vi "ard write read.vi"(8 "error in (no error)":errorcluster, 11 "VISA Refnum in":refnum<visa-resource-name>) -> (0 "error out":errorcluster, 2 "Numeric":dbl, 3 "VISA Refnum out":refnum<visa-resource-name>)   [LabVIEW 2022 SP3, in "pm Acquisition.lvlib"]
uses:
  pm Acquisition.lvlib
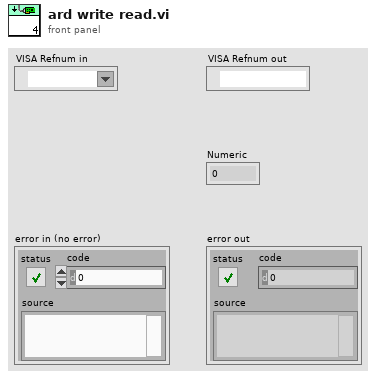
[diagram p1: front panel]
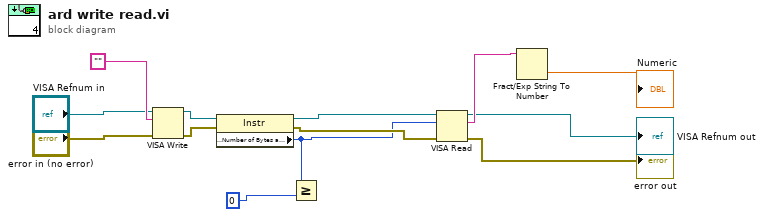
[diagram p0: block diagram]
diagram:
  n1 = VISA Write(VISA resource name="VISA Refnum in", write buffer="", error in (no error)="error in (no error)") -> (VISA resource name out=w4:refnum<visa-resource-name>, error out=w5:errorcluster)  [unwired: 1 out]
  n2 = property class="Instr"(reference=w4, error in=w5) -> (reference out=w9:refnum<visa-resource-name>, error out=w8:errorcluster, "Serial Settings:Number of Bytes at Serial Port"=w6:u32)
  n3 = Greater Or Equal?(x=w6, y=0) -> ()  [unwired: 1 out]
  n4 = VISA Read(VISA resource name=w9, byte count=w6, error in (no error)=w8) -> (VISA resource name out=→"VISA Refnum out":refnum<visa-resource-name>, read buffer=w12:string, error out=→"error out":errorcluster)  [unwired: 1 out]
  n5 = Fract/Exp String To Number(string=w12) -> (number=→"Numeric":dbl)  [unwired: 3 in, 1 out]
